vi "TIC_rw.vi"(3 "error in (no error)":errorcluster, 4 "write buffer":string, 5 "TIC 500":refnum<visa-resource-name>="COM6") -> (0 "error out":errorcluster, 1 "read buffer":string="\r\n", 2 "VISA resource name out":refnum<visa-resource-name>="COM6")   [LabVIEW 2011]
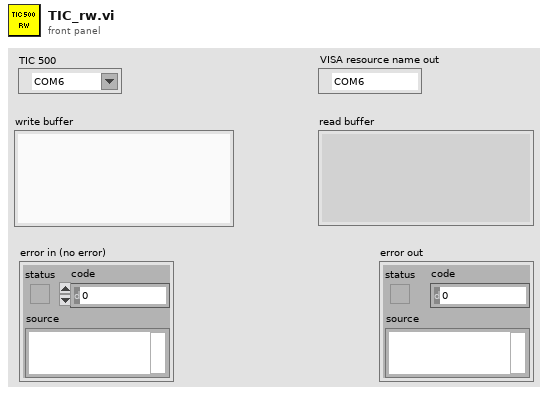
[diagram p1: front panel]
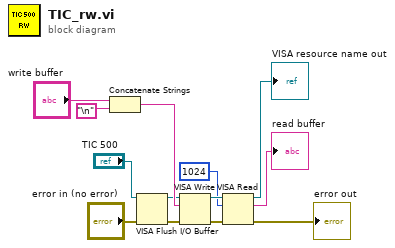
[diagram p0: block diagram]
diagram:
  n1 = Concatenate Strings("write buffer", "\n") -> (w10:string)
  n2 = VISA Flush I/O Buffer(VISA resource name="TIC 500", error in (no error)="error in (no error)") -> (VISA resource name out=w8:refnum<visa-resource-name>, error out=w6:errorcluster)  [unwired: 1 in]
  n3 = VISA Write(VISA resource name=w8, write buffer=w10, error in (no error)=w6) -> (VISA resource name out=w5:refnum<visa-resource-name>, error out=w4:errorcluster)  [unwired: 1 out]
  n4 = VISA Read(VISA resource name=w5, byte count=u32 1024, error in (no error)=w4) -> (VISA resource name out=→"VISA resource name out":refnum<visa-resource-name>, read buffer=→"read buffer":string, error out=→"error out":errorcluster)  [unwired: 1 out]
